vi "Parse Brass Matrix ERD.vi"(0 "string":string) -> (14 "Folding":i32, 16 "Jerk":i32, 18 "Jerk Delta":i32)   [LabVIEW 2021]
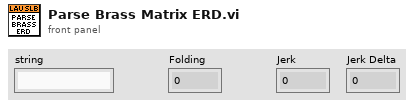
[diagram p1: front panel]
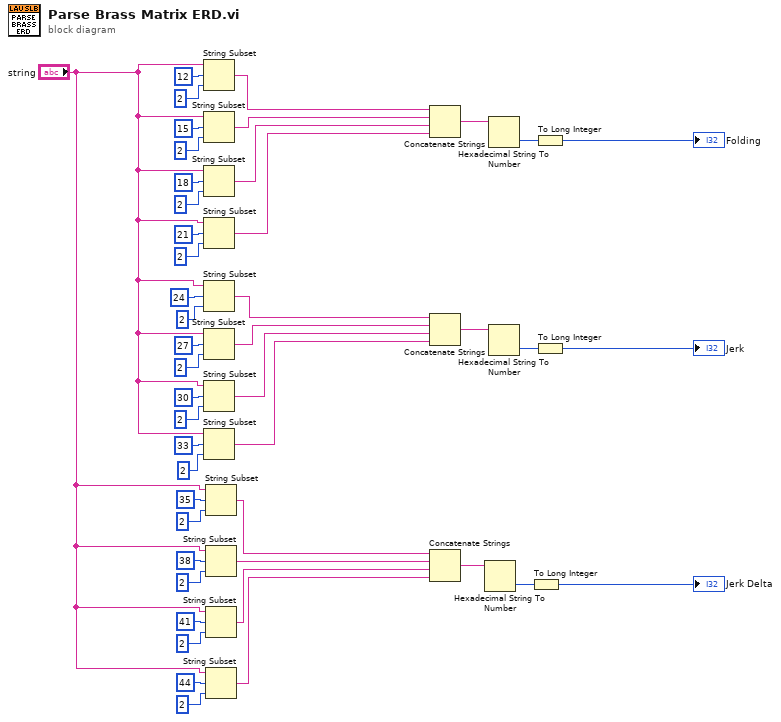
[diagram p0: block diagram]
diagram:
  n1 = String Subset(string="string", offset (0)=12, length (rest)=2 ("length (rest)")) -> (substring=w28:string)
  n2 = String Subset(string="string", offset (0)=15, length (rest)=2 ("length (rest)")) -> (substring=w27:string)
  n3 = String Subset(string="string", offset (0)=18, length (rest)=2 ("length (rest)")) -> (substring=w26:string)
  n4 = String Subset(string="string", offset (0)=21, length (rest)=2 ("length (rest)")) -> (substring=w25:string)
  n5 = String Subset(string="string", offset (0)=24, length (rest)=2 ("length (rest)")) -> (substring=w21:string)
  n6 = String Subset(string="string", offset (0)=27, length (rest)=2 ("length (rest)")) -> (substring=w20:string)
  n7 = String Subset(string="string", offset (0)=30, length (rest)=2 ("length (rest)")) -> (substring=w19:string)
  n8 = String Subset(string="string", offset (0)=33, length (rest)=2 ("length (rest)")) -> (substring=w18:string)
  n9 = String Subset(string="string", offset (0)=35, length (rest)=2 ("length (rest)")) -> (substring=w15:string)
  n10 = String Subset(string="string", offset (0)=38, length (rest)=2 ("length (rest)")) -> (substring=w14:string)
  n11 = String Subset(string="string", offset (0)=41, length (rest)=2 ("length (rest)")) -> (substring=w13:string)
  n12 = String Subset(string="string", offset (0)=44, length (rest)=2 ("length (rest)")) -> (substring=w12:string)
  n13 = Concatenate Strings(w28, w27, w26, w25) -> (w29:string)
  n14 = Concatenate Strings(w21, w20, w19, w18) -> (w23:string)
  n15 = Concatenate Strings(w15, w14, w13, w12) -> (w10:string)
  n16 = Hexadecimal String To Number(string=w10) -> (number=w11:u32)  [unwired: 2 in, 1 out]
  n17 = Hexadecimal String To Number(string=w29) -> (number=w30:u32)  [unwired: 2 in, 1 out]
  n18 = Hexadecimal String To Number(string=w23) -> (number=w22:u32)  [unwired: 2 in, 1 out]
  n19 = To Long Integer(number=w11) -> (32bit integer=→"Jerk Delta":i32)
  n20 = To Long Integer(number=w30) -> (32bit integer=→"Folding":i32)
  n21 = To Long Integer(number=w22) -> (32bit integer=→"Jerk":i32)
